vi "catchErrors.vi"(8 "error in (no error)":errorcluster, 10 "Path":path, 11 "Compiler in":refnum<class "Compiler.lvclass">) -> (0 "error out":errorcluster, 3 "Compiler out":refnum<class "Compiler.lvclass">)   [LabVIEW 2009, in "Compiler.lvlib" / "Compiler.lvclass"]
uses:
  Compiler.lvclass
  <vilib>/Utility/error.llb/DialogType.ctl
  Compiler.lvclass/Compiler.ctl
  Hal/HWController/HWControllerEvents/HWControllerEvents.lvclass
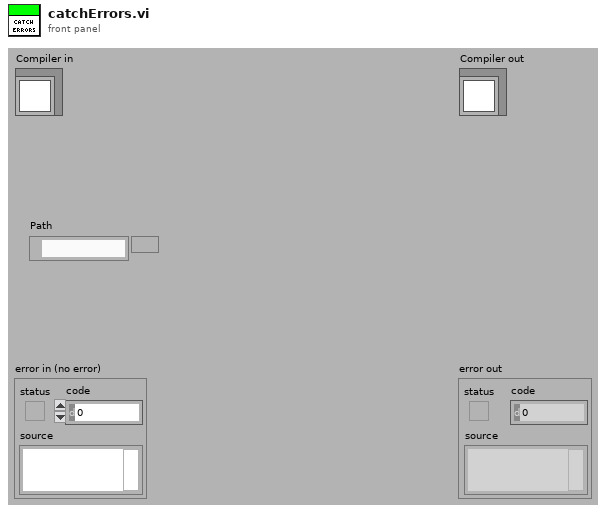
[diagram p1: front panel]
types:
  T1 = enum16{"start", "stop", "statusInquiry", "configure", "resetError", "resourcesInquiry", "reserveResources", "initialise", "resetAllChannels", "staticUpdate", "close", "HWStatus", "error", "resourcesAvailable", "resourcesReserved", "compilerError", "compiledScript", "compilingScript", "runScript", "configureCompiledScript"}
  T2 = typedef "DialogType.ctl" = u16
  T3 = cluster{"incomingEventTypes":cluster{"start":cluster{"Boolean":bool}, "stop":cluster{"Boolean":bool}, "statusInquiry":cluster{"Boolean":bool}, "configure":cluster{"DPScriptPath":path, "TimeStamp":string, "HWLoop?":bool}, "resetError":cluster{"Boolean":bool}, "resourcesInquiry":cluster{"Boolean":bool}, "reserveResources":cluster{"HWList":string[]}, "initialise":cluster{"HWList":string[]}, "close":cluster{"Boolean":bool}, "resetAllChannels":cluster{"Boolean":bool}, "staticChannelUpdate":cluster{"channel_address":string, "calibratedValue":dbl}, "runScript":cluster{"DPScriptPath":path, "TimeStamp":string, "HWLoop?":bool}, "compilingScript":cluster{"Path":path}, "compiledScript":cluster{"Path":path, "timeCompileAt":string}, "compilerError":cluster{"Path":path}, "configureCompiledScript":cluster{"DPScriptPath":path, "TimeStamp":string, "HWLoop?":bool, "CompiledScript":cluster{"ScriptListCompiler.lvclass":refnum<class "ScriptListCompiler.lvclass">, "aoChannels":refnum<class "AnalogOutput.lvclass">[], "doChannels":refnum<class "DigitalOutput.lvclass">[], "rfChannels":refnum<class "DDSOutput.lvclass">[]}}, "restartCompiler":cluster{"restart":bool}, "staticRfChannelUpdate":cluster{"channel_address":string, "Output":cluster{"Frequency(MHz)":dbl, "Amplitude":dbl, "Phase":dbl, "OutputForm":enum16{"Sine", "Square", "Triangle", "Arbitrary"}}}, "cameraUpdate":cluster{"Camera":string, "Type":string, "settings":path}}, "outgoingEventTypes":cluster{"HWStatus":cluster{"status":enum16{"Ready", "Compiling", "Configured", "Running", "Stopping", "Unresolved Error"}}, "error":cluster{"error out":errorcluster}, "resourcesAvailable":cluster{"availableHWList":string[], "reservedHWList":string[]}, "resourcesReserved":cluster{"reservedHWList":string[]}}}
  T4 = cluster{"eventId":enum16{"start", "stop", "statusInquiry", "configure", "resetError", "resourcesInquiry", "reserveResources", "initialise", "resetAllChannels", "staticUpdate", "close", "HWStatus", "error", "resourcesAvailable", "resourcesReserved", "compilerError", "compiledScript", "compilingScript", "runScript", "configureCompiledScript"}, "compilerError":cluster{"Path":path}}
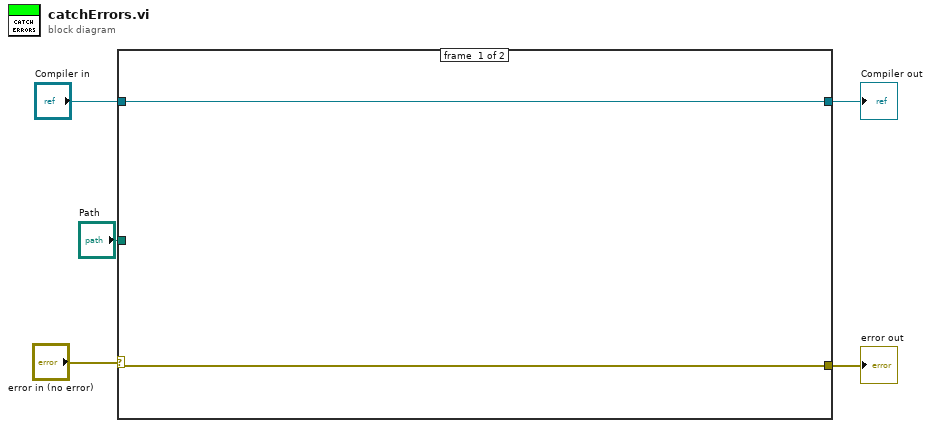
[diagram p0: block diagram]
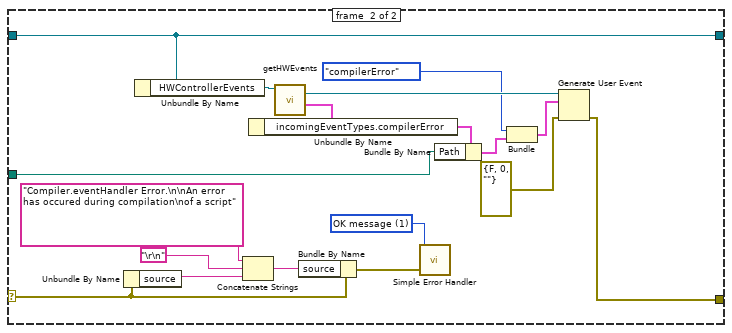
[diagram p2: hidden frame]
diagram:
  n1 = case shown="Error" "error in (no error)" {
    selector: "error in (no error)" -> [w6 w22]
    tunnel: "Compiler in" -> [w7 w24]
    tunnel: [w6 w25] -> w4
    tunnel: [w7 w24] -> w2
    tunnel: "Path" -> [_ w23]
    frame #0 {
    }
    frame #1 {
      w8 = T2 1 items=["no dialog", "OK message", "continue or stop message", "OK message + warnings", "continue/stop + warnings"] ("type of dialog (OK msg:1)")
      n2 = Unbundle By Name(w22) -> ("source"=w15:string)
      n3 = Unbundle By Name(w24) -> ("HWControllerEvents"=w21:refnum<class "HWControllerEvents.lvclass">)
      n4 = Concatenate Strings("Compiler.eventHandler Error.\n\nAn error has occured during compilation\nof a script", "\r\n", w15) -> (w11:string)
      n5 = call-dynamic "getHWEvents.vi"("HWControllerEvents in"=w21) -> ("eventDataTypes"=w20:T3, "HWCEvent"=w19:refnum<user-event>)  [unwired: 7 in, 2 out]
      n6 = Unbundle By Name(w20) -> ("incomingEventTypes.compilerError"=w16:cluster{"Path":path})
      n7 = Bundle By Name(cluster=w22, "source"=w11) -> (w9:errorcluster)
      n8 = call <vilib>:"Simple Error Handler.vi"("type of dialog (OK msg:1)"=w8, "error in (no error)"=w9) -> ()  [unwired: 3 in, 5 out]
      n9 = Bundle By Name(cluster=w16, "Path"=w23) -> (w18:cluster{"Path":path})
      n10 = Bundle("eventId"=T1."compilerError", "compilerError"=w18) -> (w17:T4)  [unwired: 1 in]
      n11 = Generate User Event(user event=w19, event data cluster=w17, error in=errorcluster {"status"=FALSE, "code"=0, "source"=""} ("output cluster")) -> (error out=w25:errorcluster)  [unwired: 1 out]
    }
  }
  "error out" <- w4
  "Compiler out" <- w2
